vi "Tester_uMsg_Delayed.vi"() -> ()   [LabVIEW 2023]
uses:
  uMsg/uMsg.lvclass
  uMsg/uMsg.lvclass/uMsg.ctl
  uMsg_Delayed.lvclass/uMsg_Delayed.ctl
  uMsg/uMsg Update Timestamp.vi
  uTransport_Event/uTransport_Event.lvclass
  U:/Projects/uFramework/Src/uFramework/uTransport/uTransport.lvclass
  uMsg_Delayed Create.vi
  uTransport/uTransport.lvclass
  uMsg_Delayed.lvclass
panel:
  in  "Msg Count":i32
  in  "Pumping Rate":i32
  in  "stop":bool
  in  "start":bool
  out "Iteration":i32
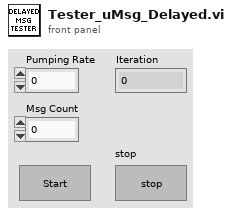
[diagram p1: front panel]
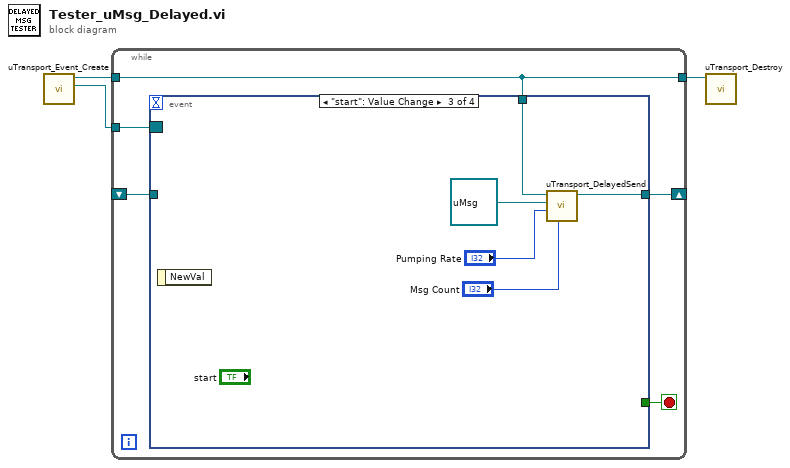
[diagram p0: block diagram]
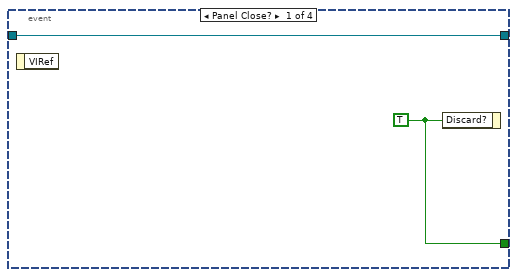
[diagram p2: hidden frame]
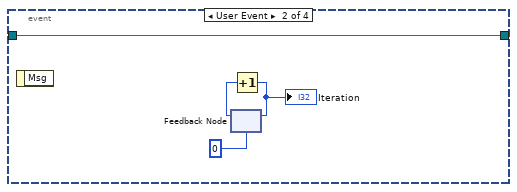
[diagram p3: hidden frame]
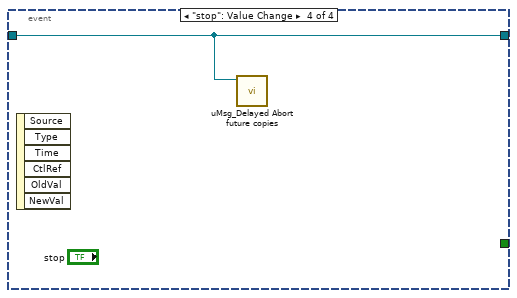
[diagram p4: hidden frame]
diagram:
  n1 = call "uTransport_Event_Create.vi"() -> ("Event:uMsg"=w1:refnum<event-registration>, "uTransport_Event out"=w2:refnum<class "uTransport_Event.lvclass">)  [unwired: 9 in, 1 out]
  n2 = while {
    tunnel: [w6] -> w3
    tunnel: w2 -> [w6]
    tunnel: w1 -> [w7]
    shift-right: [w5] -> _
    shift-left: _ -> [w4]
    stop <- w8 stop-if-true
    n3 = event shown="[2] \"start\": Value Change" {
      selector: w7 -> [_ _ _ _]
      dyn-events: _ -> [_ _ _ _]
      timeout: _ -> [_ _ _ _]
      tunnel: [w10 _ _ _] -> w8
      tunnel: w6 -> [_ _ w19 _]
      tunnel: [w9 w11 w15 w20] -> w5
      tunnel: w4 -> [w9 w11 _ w20]
      event Panel Close? {
        w10 = TRUE ("Discard?")
        n4 = event-data() -> ()  [unwired: 1 in, 1 out]
        n5 = event-data("Discard?"=w10) -> ()  [unwired: 1 in, 1 out]
      }
      event User Event {
        n6 = event-data() -> ()  [unwired: 1 in, 1 out]
        n7 = feedback #1(0) -> (w13:i32)
        n8 = Increment(x=w13) -> (x+1=w12:i32)
        "Iteration" <- w12
        n9 = feedback-in #1(w12) -> ()
      }
      event "start": Value Change {
        n10 = event-data() -> ()  [unwired: 1 in, 1 out]
        n11 = call "uTransport_DelayedSend.vi"("# of times (1)"="Msg Count", "Delay (ms)"="Pumping Rate", "Msg"=refnum<class "uMsg.lvclass"> refnum, "uTransport in"=w19) -> ("uMsg_Delayed out"=w15:refnum<class "uMsg_Delayed.lvclass">)  [unwired: 6 in, 1 out]
      }
      event "stop": Value Change {
        n12 = event-data() -> ()  [unwired: 1 in, 6 out]
        n13 = call "uMsg_Delayed Abort future copies.vi"("uMsg_Delayed in"=w20) -> ()  [unwired: 10 in, 1 out]
      }
    }
  }
  n14 = call-dynamic "uTransport_Destroy.vi"("uTransport_Event in"=w3) -> ()  [unwired: 10 in, 1 out]
